vi "Destroy.vi"(8 "Error In":errorcluster, 11 "reference in":refnum<class "ProxyImage.lvclass">) -> (0 "Error Out":errorcluster, 3 "reference out":refnum<class "ProxyImage.lvclass">)   [LabVIEW 2020, in "ProxyImage.lvclass"]
uses:
  ProxyImage.lvclass
  ProxyImage.lvclass/ProxyImage.ctl
  RealImage_class/RealImage.lvclass
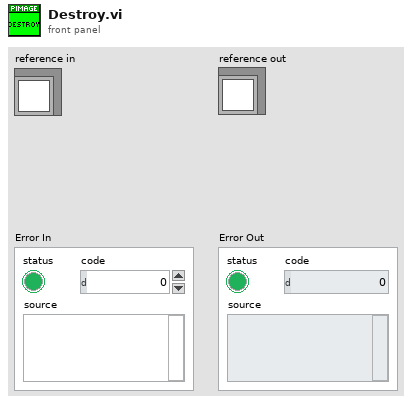
[diagram p1: front panel]
types:
  T1 = typedef "ProxyImage.lvclass/ObjectAttributes.ctl" = cluster{"_realImage":refnum<class "RealImage.lvclass">, "_fileName":string}
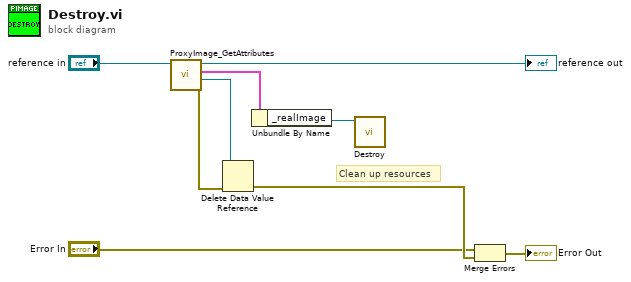
[diagram p0: block diagram]
diagram:
  # "Clean up resources"
  n1 = call "ProxyImage_GetAttributes.vi"("reference in"="reference in") -> ("error out"=w6:errorcluster, "DataRef"=w5:refnum<data-value>, "Data"=w4:T1, "reference out"=→"reference out":refnum<class "ProxyImage.lvclass">)  [unwired: 7 in]
  n2 = Delete Data Value Reference(data value reference=w5, error in=w6) -> (error out=w3:errorcluster)  [unwired: 1 out]
  n3 = Unbundle By Name(w4) -> ("_realImage"=w1:refnum<class "RealImage.lvclass">)
  n4 = call-dynamic "Destroy.vi"("reference in"=w1) -> ()  [unwired: 9 in, 2 out]
  n5 = Merge Errors("Error In", w3) -> (→"Error Out":errorcluster)
